vi "Edit.vi"(8 "error In":errorcluster, 11 "base path":path) -> (0 "error out":errorcluster, 2 "New Display":string[][](array[string]), 3 "Names List":string[](array[string])=["Ally Pulvermacher", "In", "12:30", "Initialized"])   [LabVIEW 2015]
uses:
  controls/Status.ctl
  controls/AdminStates.ctl
panel:
  in  "Status":T1 items=["", "In", "Out", "Lunch", "Break"]
  out "Time Loop Running?":bool
  out "Selected Time Stamp":string
  in  "Select Time to Add":timestamp
  in  "Okay Button":bool
  out "Employee Hours":string[][](table)
  in  "Edit In/Out":bool
  in  "Add Time":bool
  in  "Remove Time":bool
  in  "Select Employee":u16(ring) items=[" ", "Adriana Chou", "Austin Scholp", "Boquan Liu", "Colin Schrof", "David Piotrowski", "Evan Polce", "Hayley Raj", "Hunter Bourne", "Hunter Huth", "Jack Ersbo", "Jacob Tangney", "Jake Reiss", "Jennifer German", "Jessica Wang", "JJ Lamb", "Lifan Yu", "Wyatt Barber"]
  in  "Name to be added":string
  in  "Select Name":u16(ring) items=[" ", "Adriana Chou", "Austin Scholp", "Boquan Liu", "Colin Schrof", "David Piotrowski", "Evan Polce", "Hayley Raj", "Hunter Bourne", "Hunter Huth", "Jack Ersbo", "Jacob Tangney", "Jake Reiss", "Jennifer German", "Jessica Wang", "JJ Lamb", "Lifan Yu", "Wyatt Barber"]
  in  "Add Button":bool
  in  "Remove Button":bool
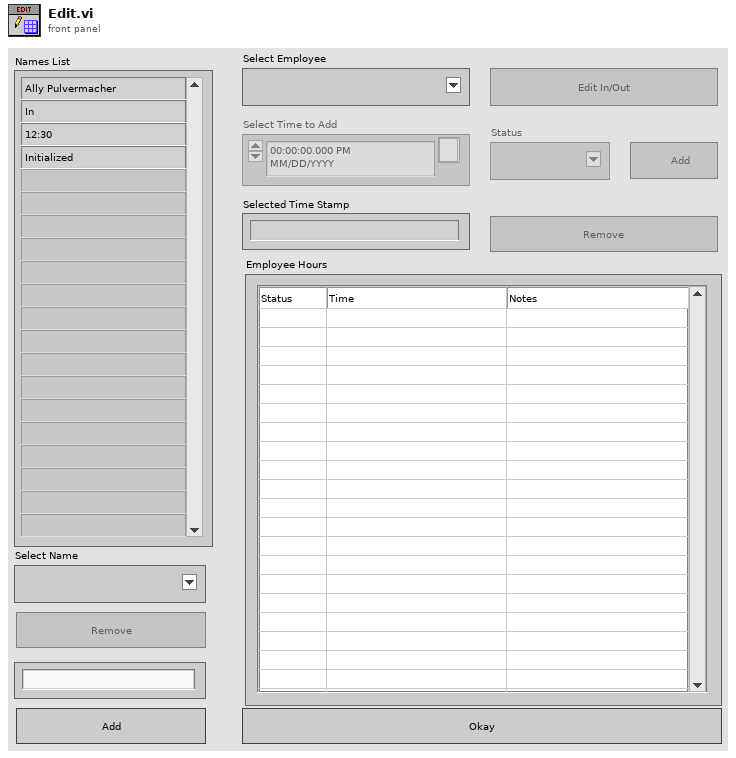
[diagram p1: front panel]
types:
  T1 = typedef "Status.ctl" = u16
  T2 = typedef "AdminStates.ctl" = enum16{"Set Display", "Wait", "Add Name", "Remove Name", "Edit In/Out", "Remove Input", "Add Input", "Exit"}
  T3 = enum8{"Enabled", "Disabled", "Disabled and Grayed Out"}
  T4 = enum16{"open", "replace", "create", "open or create", "replace or create", "replace or create with confirmation"}
  T5 = typedef "LVPoint32TypeDef.ctl" = cluster{"Horizontal":i32, "Vertical":i32}
  T6 = typedef "LVRowAndColumnTypeDef.ctl" = cluster{"Row":i32, "Column":i32}
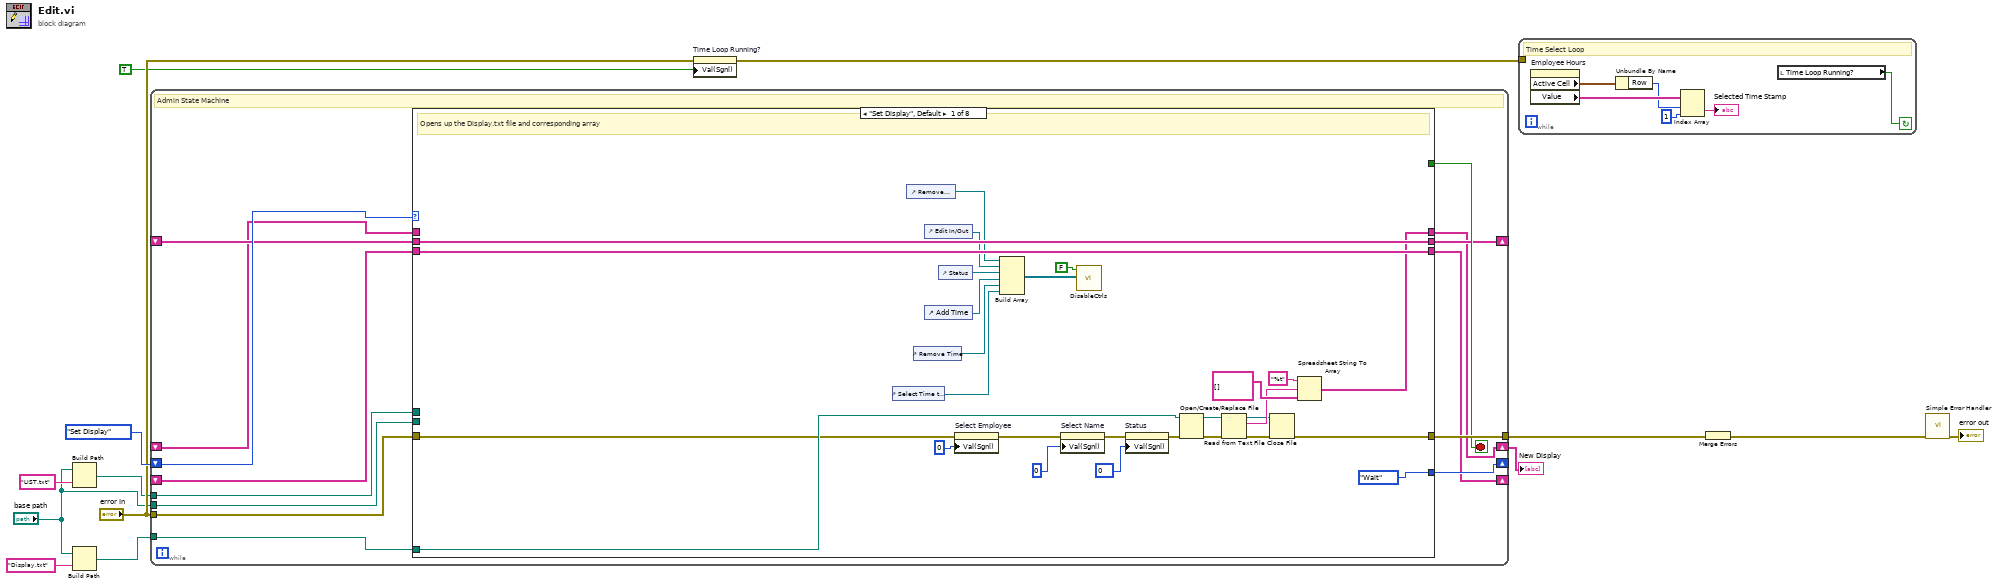
[diagram p0: block diagram]
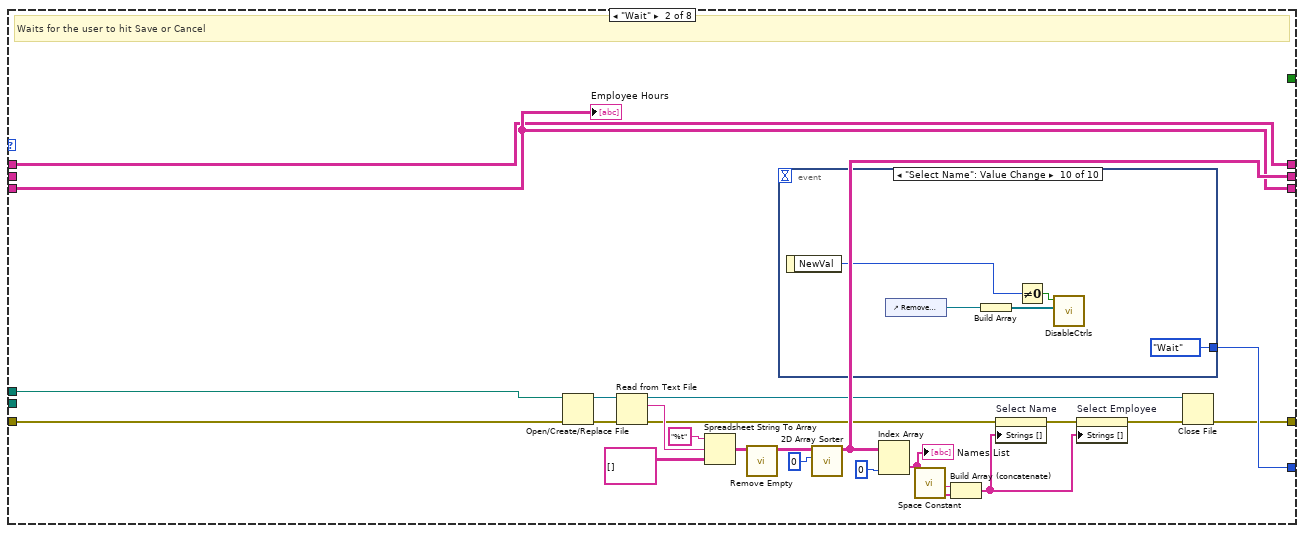
[diagram p2: hidden frame]
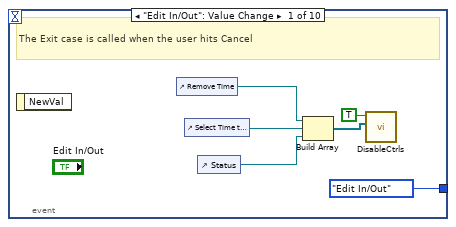
[diagram p3: hidden frame]
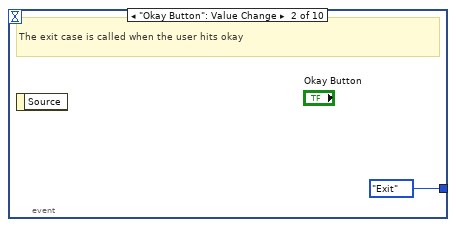
[diagram p4: hidden frame]
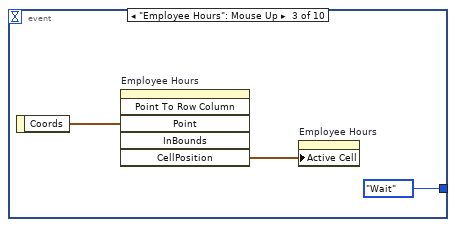
[diagram p5: hidden frame]
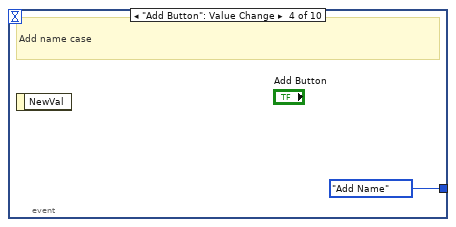
[diagram p6: hidden frame]
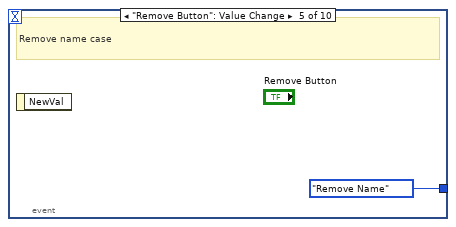
[diagram p7: hidden frame]
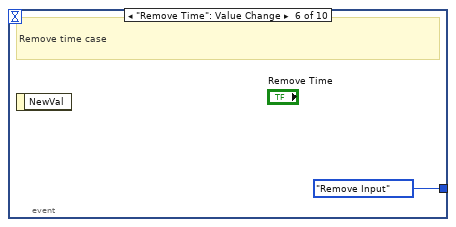
[diagram p8: hidden frame]
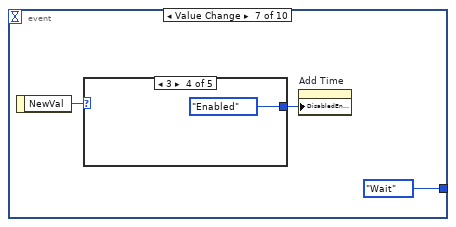
[diagram p9: hidden frame]
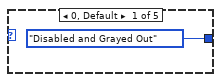
[diagram p10: hidden frame]
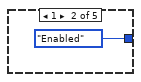
[diagram p11: hidden frame]
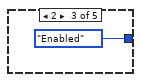
[diagram p12: hidden frame]
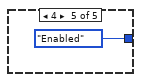
[diagram p13: hidden frame]
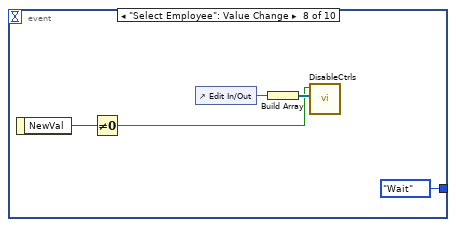
[diagram p14: hidden frame]
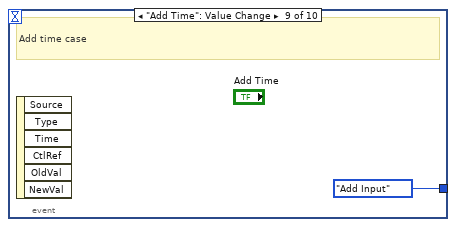
[diagram p15: hidden frame]
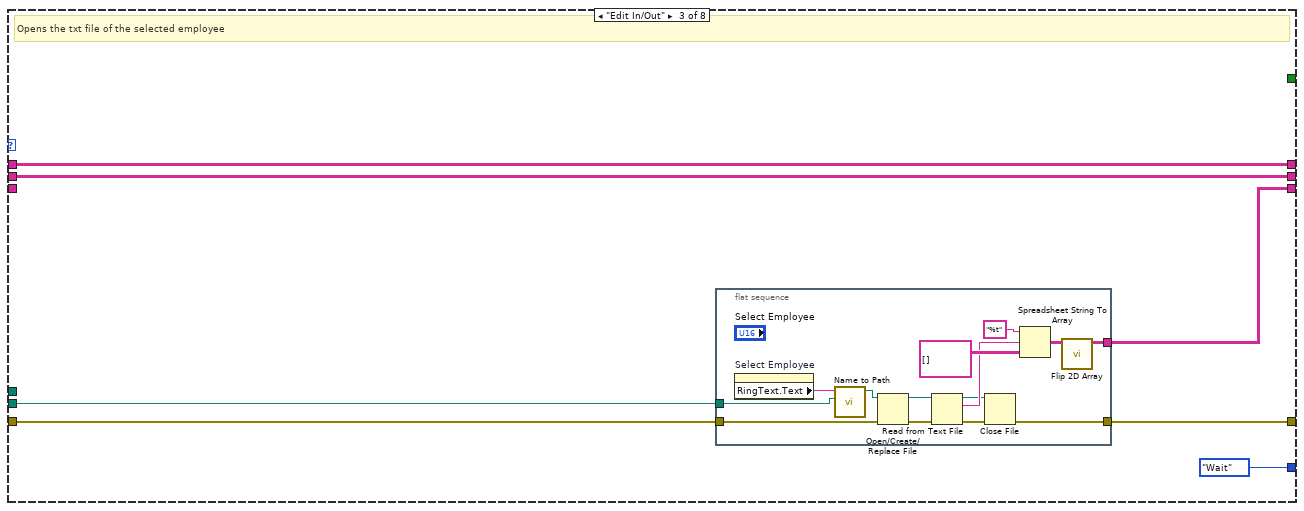
[diagram p16: hidden frame]
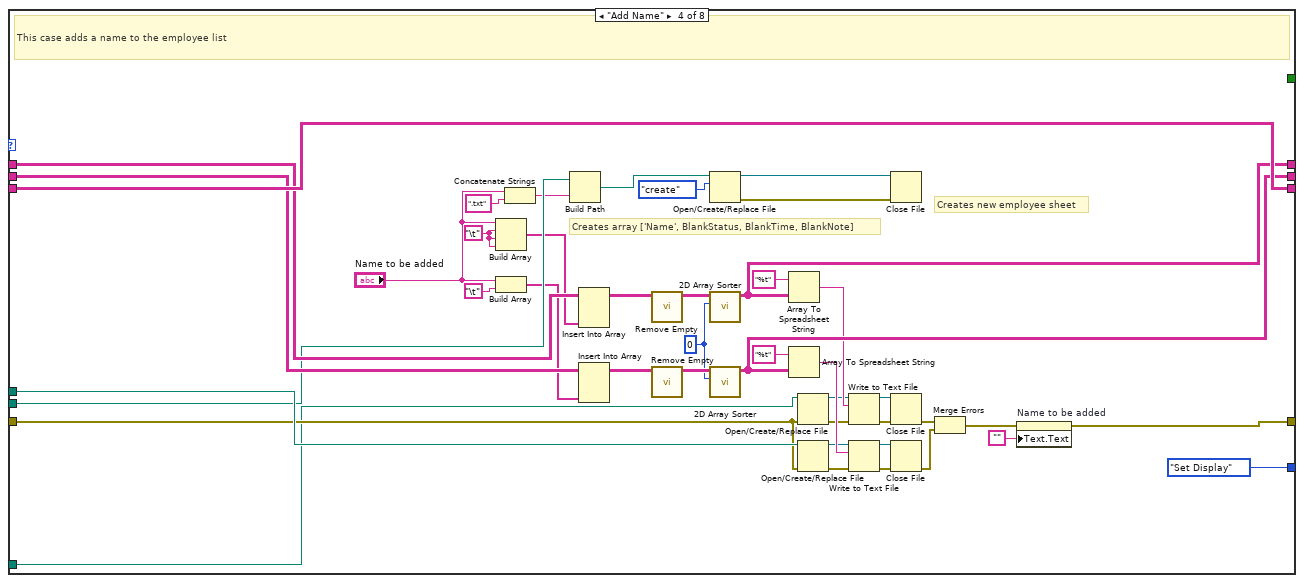
[diagram p17: hidden frame]
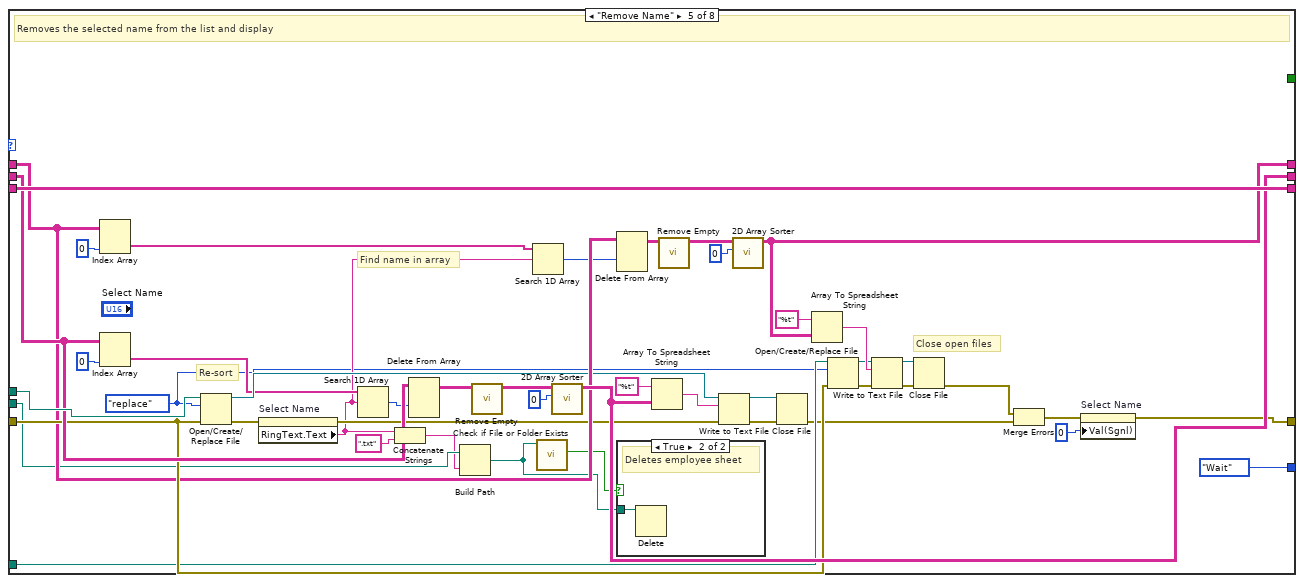
[diagram p18: hidden frame]
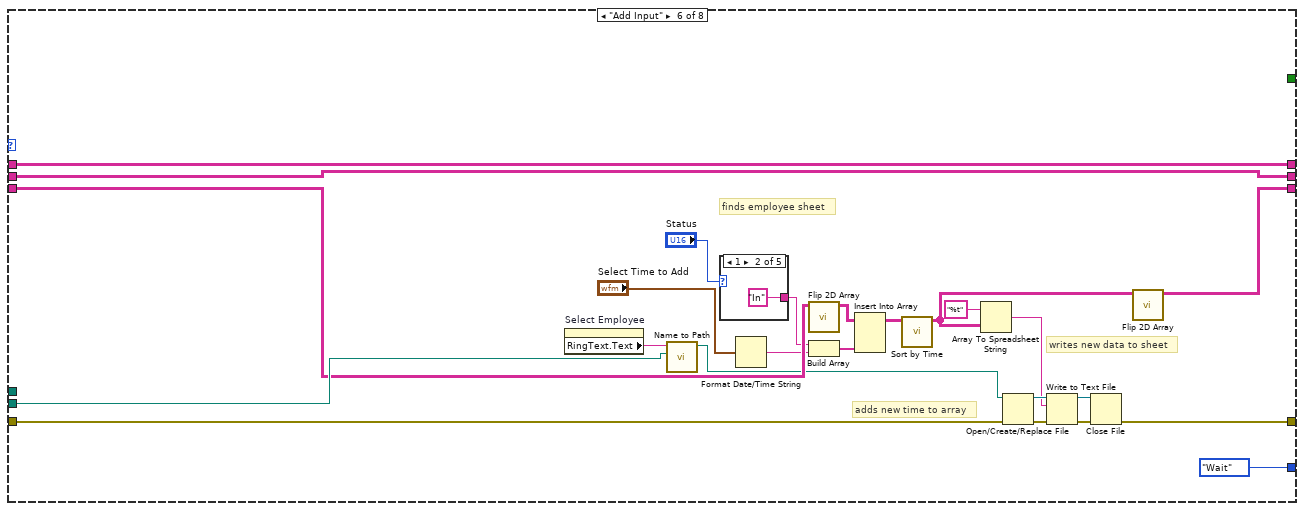
[diagram p20: hidden frame]
diagram:
  n1 = Build Path(base path="base path", name or relative path="LIST.txt") -> (appended path=w3:path)
  n2 = Build Path(base path="base path", name or relative path="Display.txt") -> (appended path=w2:path)
  n3 = while {
    tunnel: "error In" -> [w26]
    tunnel: [w25] -> w12
    shift-right: [w24] -> _
    shift-left: AdminStates."Set Display" -> [w27]
    shift-right: [w22] -> _
    shift-left: _ -> [w17]
    shift-right: [w21] -> _
    shift-left: _ -> [w20]
    tunnel: w3 -> [w19]
    tunnel: w2 -> [w18]
    shift-right: [w16] -> w6
    shift-left: _ -> [w15]
    tunnel: "base path" -> [w14]
    stop <- w23 stop-if-true
    # "Admin State Machine"
    n4 = case shown="\"Set Display\", Default" w27 {
      tunnel: w26 -> [w49 w76 w116 w166 w215 w244 w272 w283]
      tunnel: [w52 w77 w115 w171 w210 w243 w271 w283] -> w25
      tunnel: [AdminStates."Wait" w78 AdminStates."Wait" AdminStates."Set Display" AdminStates."Wait" AdminStates."Wait" AdminStates."Wait" AdminStates."Exit"] -> w24
      tunnel: [_ _ _ _ _ _ _ TRUE] -> w23
      tunnel: w19 -> [_ w75 _ w172 w218 _ _ _]
      tunnel: [w54 w73 w113 w173 w219 w238 w269 w284] -> w22
      tunnel: w17 -> [w54 w73 _ w173 w219 w239 _ w284]
      tunnel: [w53 w74 w114 w170 w217 w242 w270 w282] -> w21
      tunnel: w20 -> [w53 _ w114 w169 w216 w242 w270 w282]
      tunnel: w18 -> [w50 _ _ w165 w214 _ _ _]
      tunnel: [w51 w72 w112 w167 w212 w241 w268 w280] -> w16
      tunnel: w15 -> [_ w72 w112 w168 w213 w241 w268 w280]
      tunnel: w14 -> [_ _ w111 w164 w211 w240 w267 _]
      frame "Set Display", Default {
        w33 = T1 0 items=["", "In", "Out", "Lunch", "Break"] ("Value (Signaling)")
        # "Opens up the Display.txt file and corresponding array"
        n5 = control-ref of="Select Time to Add"() -> (w36:refnum<vi>)
        n6 = control-ref of="Remove Button"() -> (w34:refnum<vi>)
        n7 = control-ref of="Remove Time"() -> (w37:refnum<vi>)
        n8 = control-ref of="Edit In/Out"() -> (w40:refnum<vi>)
        n9 = control-ref of="Add Time"() -> (w38:refnum<vi>)
        n10 = control-ref of="Status"() -> (w39:refnum<vi>)
        n11 = property on="Select Employee" class="Ring (strict)"(error in=w49, "Val(Sgnl)"=u16 0 ("Value (Signaling)")) -> (error out=w28:errorcluster)  [unwired: 1 in, 1 out]
        n12 = Build Array(w34, w40, w39, w38, w37, w36) -> (w35:refnum<vi>[])
        n13 = property on="Select Name" class="Ring (strict)"(error in=w28, "Val(Sgnl)"=u16 0 ("Value (Signaling)")) -> (error out=w29:errorcluster)  [unwired: 1 in, 1 out]
        n14 = call "DisableCtrls.vi"("Array"=w35, "Enabled?"=FALSE ("s")) -> ()  [unwired: 10 in]
        n15 = property on="Status" class="Ring (strict)"(error in=w29, "Val(Sgnl)"=w33) -> (error out=w30:errorcluster)  [unwired: 1 in, 1 out]
        n16 = Open/Create/Replace File(file path (use dialog)=w50, error in=w30) -> (refnum out=w43:refnum<file>, error out=w45:errorcluster)  [unwired: 4 in, 1 out]
        n17 = Read from Text File(file (use dialog)=w43, error in=w45) -> (refnum out=w42:refnum<file>, text=w46:string, error out=w44:errorcluster)  [unwired: 2 in, 1 out]
        n18 = Close File(refnum=w42, error in=w44) -> (error out=w52:errorcluster)  [unwired: 1 out]
        n19 = Spreadsheet String To Array(format string="%t", spreadsheet string=w46, array type (2D Dbl)=string[][] []) -> (array=w51:string[][])  [unwired: 1 in]
      }
      frame "Wait" {
        # "Waits for the user to hit Save or Cancel"
        n20 = Open/Create/Replace File(file path (use dialog)=w75, error in=w76) -> (refnum out=w67:refnum<file>, error out=w64:errorcluster)  [unwired: 4 in, 1 out]
        n21 = Read from Text File(file (use dialog)=w67, error in=w64) -> (refnum out=w65:refnum<file>, text=w70:string, error out=w68:errorcluster)  [unwired: 2 in, 1 out]
        n22 = Spreadsheet String To Array(format string="%t", spreadsheet string=w70, array type (2D Dbl)=string[][] []) -> (array=w61:string[][])  [unwired: 1 in]
        n23 = call "Remove Empty.vi"("array in"=w61) -> ("sorted array out"=w60:string[][])  [unwired: 10 in]
        n24 = event shown="[9] \"Select Name\": Value Change" {
          selector: _ -> [_ _ _ _ _ _ _ _ _ _]
          dyn-events: _ -> [_ _ _ _ _ _ _ _ _ _]
          timeout: _ -> [_ _ _ _ _ _ _ _ _ _]
          tunnel: [AdminStates."Edit In/Out" AdminStates."Exit" AdminStates."Wait" AdminStates."Add Name" AdminStates."Remove Name" AdminStates."Remove Input" AdminStates."Wait" AdminStates."Wait" AdminStates."Add Input" AdminStates."Wait"] -> w78
          event "Edit In/Out": Value Change {
            # "The Exit case is called when the user hits Cancel"
            n25 = event-data() -> ()  [unwired: 1 in, 1 out]
            n26 = control-ref of="Remove Time"() -> (w79:refnum<vi>)
            n27 = control-ref of="Select Time to Add"() -> (w83:refnum<vi>)
            n28 = control-ref of="Status"() -> (w82:refnum<vi>)
            n29 = Build Array(w79, w83, w82) -> (w81:refnum<vi>[])
            n30 = call "DisableCtrls.vi"("Array"=w81, "Enabled?"=TRUE) -> ()  [unwired: 10 in]
          }
          event "Okay Button": Value Change {
            # "The exit case is called when the user hits okay"
            n31 = event-data() -> ()  [unwired: 1 in, 1 out]
          }
          event "Employee Hours": Mouse Up {
            n32 = event-data() -> ("Coords"=w88:T5)  [unwired: 1 in]
            n33 = invoke on="Employee Hours" class="Tbl (strict)" method="Point To Row Column"("Point"=w88) -> ("CellPosition"=w87:T6)  [unwired: 5 in, 5 out]
            n34 = property on="Employee Hours" class="Tbl (strict)"("Active Cell"=w87) -> ()  [unwired: 2 in, 2 out]
          }
          event "Add Button": Value Change {
            # "Add name case"
            n35 = event-data() -> ()  [unwired: 1 in, 1 out]
          }
          event "Remove Button": Value Change {
            # "Remove name case"
            n36 = event-data() -> ()  [unwired: 1 in, 1 out]
          }
          event "Remove Time": Value Change {
            # "Remove time case"
            n37 = event-data() -> ()  [unwired: 1 in, 1 out]
          }
          event Value Change {
            n38 = event-data() -> ("NewVal"=w94:T1)  [unwired: 1 in]
            n39 = case shown="3" w94 {
              tunnel: [T3."Disabled and Grayed Out" ("Disabled") T3."Enabled" ("Disabled") T3."Enabled" ("Disabled") T3."Enabled" ("Disabled") T3."Enabled" ("Disabled")] -> w93
              frame 0, Default {
              }
              frame 1 {
              }
              frame 2 {
              }
              frame 3 {
              }
              frame 4 {
              }
            }
            n40 = property on="Add Time" class="Bool"("DisabledEnum"=w93) -> ()  [unwired: 2 in, 2 out]
          }
          event "Select Employee": Value Change {
            n41 = event-data() -> ("NewVal"=w100:u16)  [unwired: 1 in]
            n42 = Not Equal To 0?(x=w100) -> (x != 0?=w101:bool)
            n43 = control-ref of="Edit In/Out"() -> (w103:refnum<vi>)
            n44 = Build Array(w103) -> (w102:refnum<vi>[])
            n45 = call "DisableCtrls.vi"("Array"=w102, "Enabled?"=w101) -> ()  [unwired: 10 in]
          }
          event "Add Time": Value Change {
            # "Add time case"
            n46 = event-data() -> ()  [unwired: 1 in, 6 out]
          }
          event "Select Name": Value Change {
            n47 = event-data() -> ("NewVal"=w109:u16)  [unwired: 1 in]
            n48 = control-ref of="Remove Button"() -> (w107:refnum<vi>)
            n49 = Build Array(w107) -> (w106:refnum<vi>[])
            n50 = Not Equal To 0?(x=w109) -> (x != 0?=w108:bool)
            n51 = call "DisableCtrls.vi"("Array"=w106, "Enabled?"=w108) -> ()  [unwired: 10 in]
          }
        }
        n52 = call "2D Array Sorter.vi"("Sorting Index"=0, "Array"=w60) -> ("sorted array"=w74:string[][])  [unwired: 8 in]
        n53 = Index Array(array=w74, index (col)=0 ("disabled index (col)")) -> (element=w56:string[])  [unwired: 1 in]
        "Names List" <- w56
        n54 = call <vilib>:"Space Constant.vi"() -> ("String"=w57:string)
        n55 = Build Array (concatenate)(w57, w56) -> (w58:string[])
        n56 = property on="Select Name" class="Ring (strict)"(error in=w68, "Strings []"=w58) -> (error out=w69:errorcluster)  [unwired: 1 in, 1 out]
        n57 = property on="Select Employee" class="Ring (strict)"(error in=w69, "Strings []"=w58) -> (error out=w66:errorcluster)  [unwired: 1 in, 1 out]
        n58 = Close File(refnum=w65, error in=w66) -> (error out=w77:errorcluster)  [unwired: 1 out]
        "Employee Hours" <- w73
      }
      frame "Edit In/Out" {
        # "Opens the txt file of the selected employee"
        n59 = flat-sequence {
          tunnel: w116 -> [w131]
          tunnel: [w122] -> w115
          tunnel: [w119] -> w113
          tunnel: w111 -> [w118]
          frame #0 {
            n60 = property on="Select Employee" class="Ring (strict)"() -> ("RingText.Text"=w130:string)  [unwired: 2 in, 2 out]
            n61 = call "Name to Path.vi"("Employee Sheets Path"=w118, "Employee Name"=w130) -> ("Sheet Path"=w129:path)  [unwired: 9 in]
            n62 = Open/Create/Replace File(file path (use dialog)=w129, error in=w131) -> (refnum out=w127:refnum<file>, error out=w128:errorcluster)  [unwired: 4 in, 1 out]
            n63 = Read from Text File(file (use dialog)=w127, error in=w128) -> (refnum out=w121:refnum<file>, text=w124:string, error out=w123:errorcluster)  [unwired: 2 in, 1 out]
            n64 = Close File(refnum=w121, error in=w123) -> (error out=w122:errorcluster)  [unwired: 1 out]
            n65 = Spreadsheet String To Array(format string="%t", spreadsheet string=w124, array type (2D Dbl)=string[][] []) -> (array=w120:string[][])  [unwired: 1 in]
            n66 = call "Flip 2D Array.vi"("Hours"=w120) -> ("Hours Flipped"=w119:string[][])  [unwired: 10 in]
          }
        }
      }
      frame "Add Name" {
        w132 = 0 ("index (col)")
        w146 = "\t"
        # "Creates new employee sheet"
        # "Creates array ['Name', BlankStatus, BlankTime, BlankNote]"
        # "This case adds a name to the employee list"
        n67 = Build Array("Name to be added", w146, w146, w146) -> (w145:string[])
        n68 = Build Array("Name to be added", "\t") -> (w156:string[])
        n69 = Concatenate Strings("Name to be added", ".txt" ("string")) -> (w139:string)
        n70 = Build Path(base path=w164, name or relative path=w139) -> (appended path=w138:path)
        n71 = Insert Into Array(array=w168, new element=w145) -> (w147:string[][])  [unwired: 2 in]
        n72 = Insert Into Array(array=w169, new element=w156) -> (w153:string[][])  [unwired: 2 in]
        n73 = call "Remove Empty.vi"("array in"=w147) -> ("sorted array out"=w152:string[][])  [unwired: 10 in]
        n74 = call "Remove Empty.vi"("array in"=w153) -> ("sorted array out"=w154:string[][])  [unwired: 10 in]
        n75 = Open/Create/Replace File(file path (use dialog)=w138, operation (0:open)=T4."create") -> (refnum out=w136:refnum<file>, error out=w135:errorcluster)  [unwired: 4 in, 1 out]
        n76 = call "2D Array Sorter.vi"("Sorting Index"=w132, "Array"=w152) -> ("sorted array"=w167:string[][])  [unwired: 8 in]
        n77 = call "2D Array Sorter.vi"("Sorting Index"=w132, "Array"=w154) -> ("sorted array"=w170:string[][])  [unwired: 8 in]
        n78 = Array To Spreadsheet String(array=w167, 3:"%t" ("format string")) -> (spreadsheet string=w150:string)  [unwired: 1 in]
        n79 = Array To Spreadsheet String(array=w170, 3:"%t" ("format string")) -> (spreadsheet string=w162:string)  [unwired: 1 in]
        n80 = Open/Create/Replace File(file path (use dialog)=w165, error in=w166) -> (refnum out=w149:refnum<file>, error out=w140:errorcluster)  [unwired: 4 in, 1 out]
        n81 = Open/Create/Replace File(file path (use dialog)=w172, error in=w166) -> (refnum out=w160:refnum<file>, error out=w161:errorcluster)  [unwired: 4 in, 1 out]
        n82 = Write to Text File(file (use dialog)=w149, text=w150, error in=w140) -> (refnum out=w148:refnum<file>, error out=w141:errorcluster)  [unwired: 1 in, 1 out]
        n83 = Write to Text File(file (use dialog)=w160, text=w162, error in=w161) -> (refnum out=w158:refnum<file>, error out=w159:errorcluster)  [unwired: 1 in, 1 out]
        n84 = Close File(refnum=w136, error in=w135) -> ()  [unwired: 2 out]
        n85 = Close File(refnum=w148, error in=w141) -> (error out=w142:errorcluster)  [unwired: 1 out]
        n86 = Close File(refnum=w158, error in=w159) -> (error out=w144:errorcluster)  [unwired: 1 out]
        n87 = Merge Errors(w142, w144) -> (w143:errorcluster)
        n88 = property on="Name to be added" class="Str"(error in=w143, "Text.Text"="") -> (error out=w171:errorcluster)  [unwired: 1 in, 1 out]
      }
      frame "Remove Name" {
        w179 = T4."replace" ("operation (0:open)")
        # "Close open files"
        # "Re-sort"
        # "Find name in array"
        # "Removes the selected name from the list and display"
        n89 = Index Array(array=w213, index (col)=0) -> (element=w194:string[])  [unwired: 1 in]
        n90 = Index Array(array=w216, index (col)=0 ("disabled index (col)")) -> (element=w201:string[])  [unwired: 1 in]
        n91 = Open/Create/Replace File(file path (use dialog)=w218, error in=w215, operation (0:open)=w179) -> (refnum out=w206:refnum<file>, error out=w207:errorcluster)  [unwired: 3 in, 1 out]
        n92 = property on="Select Name" class="Ring (strict)"(error in=w207) -> (error out=w203:errorcluster, "RingText.Text"=w182:string)  [unwired: 1 in, 1 out]
        n93 = Search 1D Array(1D array=w201, element=w182) -> (index of element=w197:i32)  [unwired: 1 in]
        n94 = Concatenate Strings(w182, ".txt" ("string")) -> (w184:string)
        n95 = Delete From Array(array=w216, index (row)=w197) -> (array with subset deleted=w199:string[][])  [unwired: 2 in, 1 out]
        n96 = Build Path(base path=w211, name or relative path=w184) -> (appended path=w180:path)
        n97 = call "Remove Empty.vi"("array in"=w199) -> ("sorted array out"=w200:string[][])  [unwired: 10 in]
        n98 = Search 1D Array(1D array=w194, element=w182) -> (index of element=w195:i32)  [unwired: 1 in]
        n99 = call <vilib>:"Check if File or Folder Exists.vi"("path"=w180) -> ("file or folder exists?"=w181:bool)  [unwired: 8 in, 2 out]
        n100 = call "2D Array Sorter.vi"("Sorting Index"=0, "Array"=w200) -> ("sorted array"=w217:string[][])  [unwired: 8 in]
        n101 = Delete From Array(array=w213, index (row)=w195) -> (array with subset deleted=w193:string[][])  [unwired: 2 in, 1 out]
        n102 = case shown="True" w181 {
          tunnel: w180 -> [_ w221]
          frame False {
          }
          frame True {
            # "Deletes employee sheet"
            n103 = Delete(path (use dialog)=w221) -> ()  [unwired: 4 in, 3 out]
          }
        }
        n104 = Array To Spreadsheet String(array=w217, 3:"%t" ("format string")) -> (spreadsheet string=w208:string)  [unwired: 1 in]
        n105 = call "Remove Empty.vi"("array in"=w193) -> ("sorted array out"=w192:string[][])  [unwired: 10 in]
        n106 = Write to Text File(file (use dialog)=w206, text=w208, error in=w203) -> (refnum out=w204:refnum<file>, error out=w205:errorcluster)  [unwired: 1 in, 1 out]
        n107 = call "2D Array Sorter.vi"("Sorting Index"=0, "Array"=w192) -> ("sorted array"=w212:string[][])  [unwired: 8 in]
        n108 = Close File(refnum=w204, error in=w205) -> (error out=w198:errorcluster)  [unwired: 1 out]
        n109 = Array To Spreadsheet String(array=w212, 3:"%t" ("format string")) -> (spreadsheet string=w187:string)  [unwired: 1 in]
        n110 = Open/Create/Replace File(file path (use dialog)=w214, error in=w215, operation (0:open)=w179) -> (refnum out=w186:refnum<file>, error out=w189:errorcluster)  [unwired: 3 in, 1 out]
        n111 = Write to Text File(file (use dialog)=w186, text=w187, error in=w189) -> (refnum out=w185:refnum<file>, error out=w190:errorcluster)  [unwired: 1 in, 1 out]
        n112 = Close File(refnum=w185, error in=w190) -> (error out=w191:errorcluster)  [unwired: 1 out]
        n113 = Merge Errors(w191, w198) -> (w177:errorcluster)
        n114 = property on="Select Name" class="Ring (strict)"(error in=w177, "Val(Sgnl)"=u16 0 ("Value (Signaling)")) -> (error out=w210:errorcluster)  [unwired: 1 in, 1 out]
      }
      frame "Add Input" {
        # "adds new time to array"
        # "writes new data to sheet"
        # "finds employee sheet"
        n115 = property on="Select Employee" class="Ring (strict)"() -> ("RingText.Text"=w234:string)  [unwired: 2 in, 2 out]
        n116 = call "Name to Path.vi"("Employee Sheets Path"=w240, "Employee Name"=w234) -> ("Sheet Path"=w233:path)  [unwired: 9 in]
        n117 = case shown="1" "Status" {
          tunnel: ["" ("element") "In" ("element") "Out" "Lunch" ("element") "Break" ("element")] -> w224
          frame 0, Default {
          }
          frame 1 {
          }
          frame 2 {
          }
          frame 3 {
          }
          frame 4 {
          }
        }
        n118 = Format Date/Time String(seconds (now)="Select Time to Add") -> (date/time string=w235:string)  [unwired: 2 in]
        n119 = call "Flip 2D Array.vi"("Hours"=w239) -> ("Hours Flipped"=w226:string[][])  [unwired: 10 in]
        n120 = Build Array(w224, w235) -> (w237:string[])
        n121 = Insert Into Array(array=w226, new element=w237) -> (w223:string[][])  [unwired: 2 in]
        n122 = call "Sort by Time.vi"("Sheet Array"=w223) -> ("sorted array"=w222:string[][])  [unwired: 10 in]
        n123 = Array To Spreadsheet String(array=w222, 3:"%t" ("format string")) -> (spreadsheet string=w229:string)  [unwired: 1 in]
        n124 = Open/Create/Replace File(file path (use dialog)=w233, error in=w244) -> (refnum out=w232:refnum<file>, error out=w231:errorcluster)  [unwired: 4 in, 1 out]
        n125 = Write to Text File(file (use dialog)=w232, text=w229, error in=w231) -> (refnum out=w227:refnum<file>, error out=w228:errorcluster)  [unwired: 1 in, 1 out]
        n126 = Close File(refnum=w227, error in=w228) -> (error out=w243:errorcluster)  [unwired: 1 out]
        n127 = call "Flip 2D Array.vi"("Hours"=w222) -> ("Hours Flipped"=w238:string[][])  [unwired: 10 in]
      }
      frame "Remove Input" {
        # "Locates the row that the user selects as the one they want to remove then removes it from the hours sheet"
        n128 = property on="Employee Hours" class="Tbl (strict)"() -> ("Active Cell"=w258:T6, "Value"=w254:string[][])  [unwired: 2 in, 2 out]
        n129 = property on="Select Employee" class="Ring (strict)"() -> ("RingText.Text"=w259:string)  [unwired: 2 in, 2 out]
        n130 = Unbundle By Name(w258) -> ("Row"=w253:i32)
        n131 = Array Size(array=w254) -> (size(s)=w257:i32[])
        n132 = call "Name to Path.vi"("Employee Sheets Path"=w267, "Employee Name"=w259) -> ("Sheet Path"=w266:path)  [unwired: 9 in]
        n133 = Index Array(array=w257) -> (element=w256:i32)  [unwired: 1 in]
        n134 = Greater Or Equal?(x=w253, y=w256) -> (x >= y?=w255:bool)
        n135 = case shown="True" w255 {
          tunnel: w254 -> [w277 w278]
          tunnel: w253 -> [w275 _]
          tunnel: [w274 w278] -> w269
          frame False {
            # "Delete row"
            n136 = Delete From Array(array=w277, length=1, index (row)=w275) -> (array with subset deleted=w274:string[][])  [unwired: 1 in, 1 out]
            n137 = property on="Employee Hours" class="Tbl (strict)"("Value"=w274) -> ()  [unwired: 2 in, 2 out]
          }
          frame True {
            # "Selection out of bounds"
            n138 = One Button Dialog(message="No valid row selected") -> ()  [unwired: 1 in, 1 out]
          }
        }
        n139 = call "Flip 2D Array.vi"("Hours"=w269) -> ("Hours Flipped"=w251:string[][])  [unwired: 10 in]
        n140 = Array To Spreadsheet String(array=w251, 3:"%t" ("format string")) -> (spreadsheet string=w262:string)  [unwired: 1 in]
        n141 = Open/Create/Replace File(file path (use dialog)=w266, error in=w272, operation (0:open)=T4."replace") -> (refnum out=w265:refnum<file>, error out=w264:errorcluster)  [unwired: 3 in, 1 out]
        n142 = Write to Text File(file (use dialog)=w265, text=w262, error in=w264) -> (refnum out=w260:refnum<file>, error out=w261:errorcluster)  [unwired: 1 in, 1 out]
        n143 = Close File(refnum=w260, error in=w261) -> (error out=w271:errorcluster)  [unwired: 1 out]
      }
      frame "Exit" {
        # "Exits the loop."
        "Time Loop Running?" <- FALSE
      }
    }
  }
  "New Display" <- w6
  n144 = property on="Time Loop Running?" class="Bool (strict)"(error in="error In", "Val(Sgnl)"=TRUE ("Value (Signaling)")) -> (error out=w8:errorcluster)  [unwired: 1 in, 1 out]
  n145 = while {
    tunnel: w8 -> [_]
    stop <- w292 continue-if-true
    # "Time Select Loop"
    n146 = property on="Employee Hours" class="Tbl (strict)"() -> ("Active Cell"=w291:T6, "Value"=w290:string[][])  [unwired: 2 in, 2 out]
    n147 = Unbundle By Name(w291) -> ("Row"=w289:i32)
    n148 = Index Array(array=w290, index (row)=w289, index (col)=1 ("disabled index (col)")) -> (element=→"Selected Time Stamp":string)
    n149 = local read "Time Loop Running?"() -> (w292:bool)
  }
  n150 = Merge Errors(w12) -> (w11:errorcluster)
  n151 = call <vilib>:"Simple Error Handler.vi"("error in (no error)"=w11) -> ("error out"=→"error out":errorcluster)  [unwired: 4 in, 4 out]
